vi "Config FX Extract.vi"(6 "Send Cmd Timout(ms)":u32=300, 8 "Error":errorcluster, 9 "CAN.Bus":string, 10 "HW Config":T1={"LiftHW Ver"=0, "CAN"={"ID Primary"=0, "Bus"="", "ID Follower"=0}, "Output"={"Type"=enum."Counter-Clockwise", "Neutral"=enum."Override to Coast", "Max"={"FWD"=1.0, "REV"=-1.0}, "Min"={"FWD"=0.0, "REV"=0.0}, "OL Ramp Rate (S)"=0.0, "Dead Band"=0.0}, "CLUp"={"Gains"={"P"=1.0, "I"=0.01, "D"=0.0, "F"=0.0}, "Error Allowed"={"High"=0.0, "Low"=0.0}, "I Zone"={"High"=10000.0, "Low"=-1000.0}, "Max Out"={"FWD"=1.0, "REV"=-1.0}, "Max I Accu"={"High"=10.0, "Low"=-10.0}, "CL Ramp Rate (S)"=0.0}, "MM"={"Cruise Velocity"=5000, "Acceleration"=5000}, "TravelLimits"={"Hard"={"FWD Switch Normal"=enum."Normally Open", "FWD On will Zero Encoder "=FALSE, "REV Switch Normal"=enum."Normally Open", "REV On will Zero Encoder "=FALSE}, "Soft"={"FWD"={"Enable"=FALSE, "Counts"=0}, "REV"={"Enable"=FALSE, "Counts"=0}}}, "Cancoder"={"ID"=0, "CW(t) CCW(f)"=TRUE, "Zero Offset"=0.0}, "CLDown"={"Gains"={"P"=1.0, "I"=0.01, "D"=0.0, "F"=0.0}, "Error Allowed"={"High"=0.0, "Low"=0.0}, "I Zone"={"High"=10000.0, "Low"=-1000.0}, "Max Out"={"FWD"=1.0, "REV"=-1.0}, "Max I Accu"={"High"=10.0, "Low"=-10.0}, "CL Ramp Rate (S)"=0.0}, "CurrentLimit"={"Enable"=FALSE, "Current Limit"=0.0, "Threshold Current"=0.0, "Threshold Time"=0.0}} {"CLDown"."Max I Accu"."Low" format="%#.8f"; "CLDown"."Max I Accu"."High" format="%#.8f"; "CLDown"."Gains"."F" format="%#.8f"; "CLDown"."Gains"."D" format="%#.8f"; "CLDown"."Gains"."I" format="%#.8f"; "CLDown"."Gains"."P" format="%#.8f"; "CLDown"."Error Allowed"."Low" format="%#.8f"; "CLDown"."Error Allowed"."High" format="%#.8f"; "CLDown"."I Zone"."Low" format="%#.8f"; "CLDown"."I Zone"."High" format="%#.8f"; "CLDown"."Max Out"."REV" format="%.2f"; "CLDown"."Max Out"."FWD" format="%.2f"; "TravelLimits"."Soft"."REV"."Counts" format="%#.0f"; "TravelLimits"."Soft"."FWD"."Counts" format="%#.0f"; "Output"."Min"."REV" format="%.2f"; "Output"."Min"."FWD" format="%.2f"; "Output"."Max"."REV" format="%.2f"; "Output"."Max"."FWD" format="%.2f"; "CLUp"."Max I Accu"."Low" format="%#.8f"; "CLUp"."Max I Accu"."High" format="%#.8f"; "CLUp"."Gains"."F" format="%#.8f"; "CLUp"."Gains"."D" format="%#.8f"; "CLUp"."Gains"."I" format="%#.8f"; "CLUp"."Gains"."P" format="%#.8f"; "CLUp"."Error Allowed"."Low" format="%#.8f"; "CLUp"."Error Allowed"."High" format="%#.8f"; "CLUp"."I Zone"."Low" format="%#.8f"; "CLUp"."I Zone"."High" format="%#.8f"; "CLUp"."Max Out"."REV" format="%.2f"; "CLUp"."Max Out"."FWD" format="%.2f"}, 11 "PhoenixMotorControlDevRef":T18={"DeviceStatus"={"status"=FALSE, "code"=0, "source"=""}, "Type"=enum."PWM", "PWM"={"PWM Channel"=enum."Invalid", "DeadBand"={"Name"="", "maxPositivePwm"=0, "minPositivePwm"=0, "centerPwm"=0, "maxNegativePwm"=0, "minNegativePwm"=0, "angularRange"=0}}, "CAN"={"Device Number"=0, "SetOutput VI Ref"=variant, "GetOutput VI Ref"=variant, "Enable VI Ref"=variant, "Disable VI Ref"=variant, "Data"=variant}, "Invert"=FALSE, "DIO PWM"={"PWM \"Enable\" Channel"=enum."Invalid", "DIOChannel"=enum."Invalid", "PWM Rate"=0.0}}) -> (0 "Error Out":errorcluster, 2 "HW Config Data Out":T1={"LiftHW Ver"=0, "CAN"={"ID Primary"=0, "Bus"="", "ID Follower"=0}, "Output"={"Type"=enum."Counter-Clockwise", "Neutral"=enum."Override to Coast", "Max"={"FWD"=1.0, "REV"=-1.0}, "Min"={"FWD"=0.0, "REV"=0.0}, "OL Ramp Rate (S)"=0.0, "Dead Band"=0.0}, "CLUp"={"Gains"={"P"=1.0, "I"=0.01, "D"=0.0, "F"=0.0}, "Error Allowed"={"High"=0.0, "Low"=0.0}, "I Zone"={"High"=10000.0, "Low"=-1000.0}, "Max Out"={"FWD"=1.0, "REV"=-1.0}, "Max I Accu"={"High"=10.0, "Low"=-10.0}, "CL Ramp Rate (S)"=0.0}, "MM"={"Cruise Velocity"=5000, "Acceleration"=5000}, "TravelLimits"={"Hard"={"FWD Switch Normal"=enum."Normally Open", "FWD On will Zero Encoder "=FALSE, "REV Switch Normal"=enum."Normally Open", "REV On will Zero Encoder "=FALSE}, "Soft"={"FWD"={"Enable"=FALSE, "Counts"=0}, "REV"={"Enable"=FALSE, "Counts"=0}}}, "Cancoder"={"ID"=0, "CW(t) CCW(f)"=TRUE, "Zero Offset"=0.0}, "CLDown"={"Gains"={"P"=1.0, "I"=0.01, "D"=0.0, "F"=0.0}, "Error Allowed"={"High"=0.0, "Low"=0.0}, "I Zone"={"High"=10000.0, "Low"=-1000.0}, "Max Out"={"FWD"=1.0, "REV"=-1.0}, "Max I Accu"={"High"=10.0, "Low"=-10.0}, "CL Ramp Rate (S)"=0.0}, "CurrentLimit"={"Enable"=FALSE, "Current Limit"=0.0, "Threshold Current"=0.0, "Threshold Time"=0.0}} {"CLDown"."Max I Accu"."Low" format="%#.8f"; "CLDown"."Max I Accu"."High" format="%#.8f"; "CLDown"."Gains"."F" format="%#.8f"; "CLDown"."Gains"."D" format="%#.8f"; "CLDown"."Gains"."I" format="%#.8f"; "CLDown"."Gains"."P" format="%#.8f"; "CLDown"."Error Allowed"."Low" format="%#.8f"; "CLDown"."Error Allowed"."High" format="%#.8f"; "CLDown"."I Zone"."Low" format="%#.8f"; "CLDown"."I Zone"."High" format="%#.8f"; "CLDown"."Max Out"."REV" format="%.2f"; "CLDown"."Max Out"."FWD" format="%.2f"; "TravelLimits"."Soft"."REV"."Counts" format="%#.0f"; "TravelLimits"."Soft"."FWD"."Counts" format="%#.0f"; "Output"."Min"."REV" format="%.2f"; "Output"."Min"."FWD" format="%.2f"; "Output"."Max"."REV" format="%.2f"; "Output"."Max"."FWD" format="%.2f"; "CLUp"."Max I Accu"."Low" format="%#.8f"; "CLUp"."Max I Accu"."High" format="%#.8f"; "CLUp"."Gains"."F" format="%#.8f"; "CLUp"."Gains"."D" format="%#.8f"; "CLUp"."Gains"."I" format="%#.8f"; "CLUp"."Gains"."P" format="%#.8f"; "CLUp"."Error Allowed"."Low" format="%#.8f"; "CLUp"."Error Allowed"."High" format="%#.8f"; "CLUp"."I Zone"."Low" format="%#.8f"; "CLUp"."I Zone"."High" format="%#.8f"; "CLUp"."Max Out"."REV" format="%.2f"; "CLUp"."Max Out"."FWD" format="%.2f"}, 3 "Module Azimuth Ref Out":T18)   [LabVIEW 2020, in "Lift_ACT.lvlib"]
uses:
  Lift_ACT.lvlib
  <vilib>/Rock Robotics/WPI/MotorControl/WPI_MotorControlDeviceRef.ctl
  <vilib>/Rock Robotics/WPI/MotorControl/WPI_MotorControlType.ctl
  <vilib>/Rock Robotics/SystemInterfaces/DIO/FPGA_DIOPWMChannel.ctl
  <vilib>/Rock Robotics/WPI/PWM/WPI_PWMDeadband.ctl
  <vilib>/Rock Robotics/SystemInterfaces/DIO/FPGA_DIOChannel.ctl
  Shared Code/TypeDefs/Cluster_Lift_Config HW Values.ctl
  Shared Code/TypeDefs/Cluser_CAN Follower Data.ctl
  Shared Code/TypeDefs/Cluster_Config Motor Output.ctl
  <vilib>/Rock Robotics/WPI/ThirdParty/Phoenix-LabVIEW/Motor Controller/Controls/CTRE_Phoenix_MotorControl_TalonFXInvertType.ctl
  <vilib>/Rock Robotics/WPI/ThirdParty/Phoenix-LabVIEW/Motor Controller/Controls/CTRE_Phoenix_MotorControl_NeutralMode.ctl
  Shared Code/TypeDefs/Cluster_FWD  REV Values.ctl
  Shared Code/TypeDefs/Cluster_PID Config.ctl
  Shared Code/TypeDefs/Cluster_PID Gains.ctl
  Shared Code/TypeDefs/Cluster_High-Low.ctl
  Shared Code/TypeDefs/Cluster_Motion Magic Parameters.ctl
  Shared Code/TypeDefs/Cluser_Limit Travel Config.ctl
  Shared Code/TypeDefs/Cluser_Hard Limits.ctl
  <vilib>/Rock Robotics/WPI/ThirdParty/Phoenix-LabVIEW/Motor Controller/Controls/CTRE_Phoenix_MotorControl_LimitSwitchNormal.ctl
  Shared Code/TypeDefs/Cluser_Config_Soft Limits.ctl
  Shared Code/TypeDefs/Cluser_Enable-Value I32.ctl
  Shared Code/TypeDefs/Cluster_Config_Cancoder Data.ctl
  Shared Code/TypeDefs/Cluser_Config_Current Limits.ctl
  <vilib>/Rock Robotics/WPI/ThirdParty/Phoenix-LabVIEW/Motor Controller/Controls/CTRE_Phoenix_MotorControl_TalonFXMotorControllerConfigurables.ctl
  <vilib>/Rock Robotics/WPI/ThirdParty/Phoenix-LabVIEW/Motor Controller/Controls/CTRE_Phoenix_MotorControl_BaseConfigurables.ctl
  <vilib>/Rock Robotics/WPI/ThirdParty/Phoenix-LabVIEW/Motor Controller/Controls/CTRE_Phoenix_MotorControl_VelocityMeasurementPeriod.ctl
  <vilib>/Rock Robotics/WPI/ThirdParty/Phoenix-LabVIEW/Motor Controller/Controls/CTRE_Phoenix_MotorControl_SlotStructure.ctl
  <vilib>/Rock Robotics/WPI/ThirdParty/Phoenix-LabVIEW/Motor Controller/Controls/CTRE_Phoenix_MotorControl_FilterStruct.ctl
  <vilib>/Rock Robotics/WPI/ThirdParty/Phoenix-LabVIEW/Motor Controller/Controls/CTRE_Phoenix_MotorControl_RemoteSourceType.ctl
  <vilib>/Rock Robotics/WPI/ThirdParty/Phoenix-LabVIEW/Controls/CTRE_Phoenix_CustomParamConfiguration.ctl
  <vilib>/Rock Robotics/WPI/ThirdParty/Phoenix-LabVIEW/Motor Controller/Controls/CTRE_Phoenix_MotorControl_FeedbackDevice_TalonFX.ctl
  <vilib>/Rock Robotics/WPI/ThirdParty/Phoenix-LabVIEW/Motor Controller/Controls/CTRE_Phoenix_MotorControl_LimitSwitchSource_Local.ctl
  <vilib>/Rock Robotics/WPI/ThirdParty/Phoenix-LabVIEW/Motor Controller/Controls/CTRE_Phoenix_MotorControl_SupplyCurrentLimitConfiguration.ctl
  <vilib>/Rock Robotics/WPI/ThirdParty/Phoenix-LabVIEW/Motor Controller/Controls/CTRE_Phoenix_MotorControl_StatorCurrentLimitConfiguration.ctl
  <vilib>/Rock Robotics/WPI/ThirdParty/Phoenix-LabVIEW/Motor Controller/Controls/CTRE_Phoenix_MotorControl_MotorCommutation_TalonFX.ctl
  <vilib>/Rock Robotics/WPI/ThirdParty/Phoenix-LabVIEW/CANCoder/Controls/CTRE_Phoenix_CANcoder_AbsoluteSensorRange.ctl
  <vilib>/Rock Robotics/WPI/ThirdParty/Phoenix-LabVIEW/CANCoder/Controls/CTRE_Phoenix_CANcoder_SensorInitializationStrategy.ctl
  <vilib>/Utility/Data Type/NI_Data Type.lvlib
panel:
  # "Tune Output\nto 1023 Max"
  # "Tune Output\nto 1023 Max"
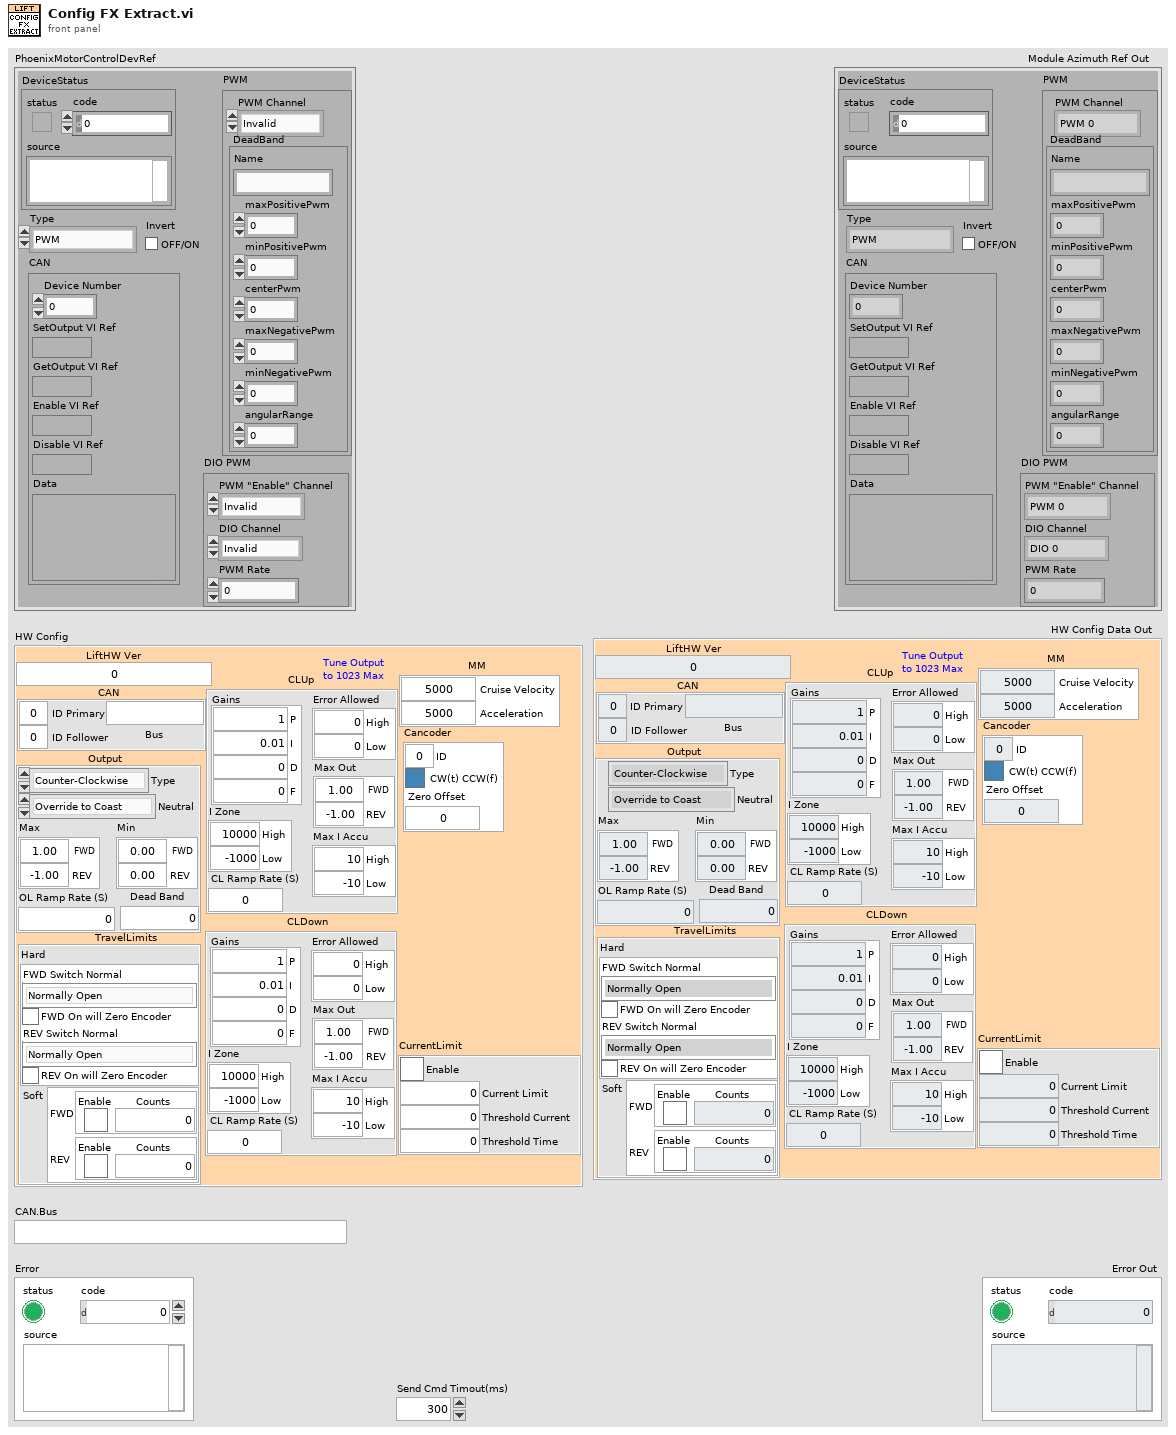
[diagram p1: front panel]
types:
  T1 = typedef "Cluster_Lift_Config HW Values.ctl" = cluster{"LiftHW Ver":u64, "CAN":T2, "Output":T3, "CLUp":T7, "MM":T10, "TravelLimits":T11, "Cancoder":T16, "CLDown":T7, "CurrentLimit":T17}
  T2 = typedef "Cluser_CAN Follower Data.ctl" = cluster{"ID Primary":u8, "Bus":string, "ID Follower":u8}
  T3 = typedef "Cluster_Config Motor Output.ctl" = cluster{"Type":T4, "Neutral":T5, "Max":T6, "Min":T6, "OL Ramp Rate (S)":dbl, "Dead Band":dbl}
  T4 = typedef "CTRE_Phoenix_MotorControl_TalonFXInvertType.ctl" = enum16{"Counter-Clockwise", "Clockwise"}
  T5 = typedef "CTRE_Phoenix_MotorControl_NeutralMode.ctl" = enum8{"EEPROMSetting", "Override to Coast", "Override to Brake"}
  T6 = typedef "Cluster_FWD  REV Values.ctl" = cluster{"FWD":dbl, "REV":dbl}
  T7 = typedef "Cluster_PID Config.ctl" = cluster{"Gains":T8, "Error Allowed":T9, "I Zone":T9, "Max Out":T6, "Max I Accu":T9, "CL Ramp Rate (S)":dbl}
  T8 = typedef "Cluster_PID Gains.ctl" = cluster{"P":dbl, "I":dbl, "D":dbl, "F":dbl}
  T9 = typedef "Cluster_High-Low.ctl" = cluster{"High":dbl, "Low":dbl}
  T10 = typedef "Cluster_Motion Magic Parameters.ctl" = cluster{"Cruise Velocity":i32, "Acceleration":i32}
  T11 = typedef "Cluser_Limit Travel Config.ctl" = cluster{"Hard":T12, "Soft":T14}
  T12 = typedef "Cluser_Hard Limits.ctl" = cluster{"FWD Switch Normal":T13, "FWD On will Zero Encoder ":bool, "REV Switch Normal":T13, "REV On will Zero Encoder ":bool}
  T13 = typedef "CTRE_Phoenix_MotorControl_LimitSwitchNormal.ctl" = enum16{"Normally Open", "Normally Closed", "Disabled"}
  T14 = typedef "Cluser_Config_Soft Limits.ctl" = cluster{"FWD":T15, "REV":T15}
  T15 = typedef "Cluser_Enable-Value I32.ctl" = cluster{"Enable":bool, "Counts":i32}
  T16 = typedef "Cluster_Config_Cancoder Data.ctl" = cluster{"ID":u8, "CW(t) CCW(f)":bool, "Zero Offset":dbl}
  T17 = typedef "Cluser_Config_Current Limits.ctl" = cluster{"Enable":bool, "Current Limit":dbl, "Threshold Current":dbl, "Threshold Time":dbl}
  T18 = typedef "WPI_MotorControlDeviceRef.ctl" = cluster{"DeviceStatus":errorcluster, "Type":T19, "PWM":cluster{"PWM Channel":T20, "DeadBand":T21}, "CAN":cluster{"Device Number":u8, "SetOutput VI Ref":variant, "GetOutput VI Ref":variant, "Enable VI Ref":variant, "Disable VI Ref":variant, "Data":variant}, "Invert":bool, "DIO PWM":cluster{"PWM \"Enable\" Channel":T20, "DIOChannel":T22, "PWM Rate":dbl}}
  T19 = typedef "WPI_MotorControlType.ctl" = enum16{"PWM", "CAN", "DIO PWM"}
  T20 = typedef "FPGA_DIOPWMChannel.ctl" = enum8{"PWM 0", "PWM 1", "PWM 2", "PWM 3", "PWM 4", "PWM 5", "PWM 6", "PWM 7", "PWM 8", "PWM 9", "PWM MXP 0", "PWM MXP 1", "PWM MXP 2", "PWM MXP 3", "PWM MXP 4", "PWM MXP 5", "PWM MXP 6", "PWM MXP 7", "PWM MXP 8", "PWM MXP 9", "Invalid"}
  T21 = typedef "WPI_PWMDeadband.ctl" = cluster{"Name":string, "maxPositivePwm":i32, "minPositivePwm":i32, "centerPwm":i32, "maxNegativePwm":i32, "minNegativePwm":i32, "angularRange":u16}
  T22 = typedef "FPGA_DIOChannel.ctl" = enum8{"DIO 0", "DIO 1", "DIO 2", "DIO 3", "DIO 4", "DIO 5", "DIO 6", "DIO 7", "DIO 8", "DIO 9", "DIO MXP 0", "DIO MXP 1", "DIO MXP 2", "DIO MXP 3", "DIO MXP 4", "DIO MXP 5", "DIO MXP 6", "DIO MXP 7", "DIO MXP 8", "DIO MXP 9", "DIO MXP 10", "DIO MXP 11", "DIO MXP 12", "DIO MXP 13", "DIO MXP 14", "DIO MXP 15", "SPI Port CS1", "SPI Port CS2", "SPI Port CS3", "SPI Port MISO", "SPI Port MOSI", "Invalid"}
  T23 = typedef "CTRE_Phoenix_MotorControl_TalonFXMotorControllerConfigurables.ctl" = cluster{"Base Configurables":T24, "primaryPID":cluster{"selectedFeedbackCoefficient":dbl, "selectedFeedbackSensor":T30}, "auxiliaryPID":cluster{"selectedFeedbackCoefficient":dbl, "selectedFeedbackSensor":T30}, "forwardLimitSwitchNormal":T13, "reverseLimitSwitchNormal":T13, "forwardLimitSwitchDeviceID":i32, "reverseLimitSwitchDeviceID":i32, "forwardLimitSwitchSource":T31, "reverseLimitSwitchSource":T31, "sum0Term":T30, "sum1Term":T30, "diff0Term":T30, "diff1Term":T30, "Supply Current Limit Configuration":T32, "Stator Current Limit Configuration":T33, "Motor Commutation":T34, "Absolute Sensor Range":T35, "Integrated Sensor Offset (Degrees)":dbl, "Sensor Initialization Strategy":T36}
  T24 = typedef "CTRE_Phoenix_MotorControl_BaseConfigurables.ctl" = cluster{"openLoopRamp":dbl, "closedLoopRamp":dbl, "peakOutputForward":dbl, "peakOutputReverse":dbl, "nominalOutputForward":dbl, "nominalOutputReverse":dbl, "neutralDeadband":dbl, "voltageCompSaturation":dbl, "voltageMeasurementFilter":i32, "velocityMeasurementPeriod":T25, "velocityMeasurementWindow":i32, "forwardSoftLimitThreshold":i32, "reverseSoftLimitThreshold":i32, "forwardSoftLimitEnable":bool, "reverseSoftLimitEnable":bool, "slot0":T26, "slot1":T26, "slot2":T26, "slot3":T26, "auxPIDPolarity":bool, "remoteFilter0":T27, "remoteFilter1":T27, "motionCruiseVelocity":i32, "motionAcceleration":i32, "motionProfileTrajectoryPeriod":i32, "feedbackNotContinuous":bool, "remoteSensorClosedLoopDisableNeutralOnLOS":bool, "clearPositionOnLimitF":bool, "clearPositionOnLimitR":bool, "clearPositionOnQuadIdx":bool, "limitSwitchDisableNeutralOnLOS":bool, "softLimitDisableNeutralOnLOS":bool, "pulseWidthPeriod_EdgesPerRot":i32, "pulseWidthPeriod_FilterWindowSz":i32, "customParam":T29, "trajectoryInterpolationEnable":bool}
  T25 = typedef "CTRE_Phoenix_MotorControl_VelocityMeasurementPeriod.ctl" = u16
  T26 = typedef "CTRE_Phoenix_MotorControl_SlotStructure.ctl" = cluster{"P":dbl, "I":dbl, "D":dbl, "F":dbl, "integralZone":dbl, "allowableClosedLoopError":i32, "maxIntegralAccumulator":dbl, "closedLoopPeakOutput":dbl, "closedLoopPeriod":i32}
  T27 = typedef "CTRE_Phoenix_MotorControl_FilterStruct.ctl" = cluster{"remoteSensorDeviceID":u8, "remoteSensorSource":T28}
  T28 = typedef "CTRE_Phoenix_MotorControl_RemoteSourceType.ctl" = enum16{"Off", "Talon SRX Selected Sensor", "Pigeon IMU Yaw", "Pigeon IMU Pitch", "Pigeon IMU Roll", "CANifier Quadrature", "CANifier PWM Input 0", "CANifier PWM Input 1", "CANifier PWM Input 2", "CANifier PWM Input 3", "Gadgeteer Pigeon Yaw", "Gadgeteer Pigeon Pitch", "Gadgeteer Pigeon Roll", "CANCoder"}
  T29 = typedef "CTRE_Phoenix_CustomParamConfiguration.ctl" = cluster{"customParam0":i32, "customParam1":i32}
  T30 = typedef "CTRE_Phoenix_MotorControl_FeedbackDevice_TalonFX.ctl" = i8
  T31 = typedef "CTRE_Phoenix_MotorControl_LimitSwitchSource_Local.ctl" = enum16{"Feedback Connector", "Remote Talon SRX", "Remote CANifier", "Deactivated"}
  T32 = typedef "CTRE_Phoenix_MotorControl_SupplyCurrentLimitConfiguration.ctl" = cluster{"Enable?":bool, "Current Limit":dbl, "Threshold Current":dbl, "Threshold Time":dbl}
  T33 = typedef "CTRE_Phoenix_MotorControl_StatorCurrentLimitConfiguration.ctl" = cluster{"Enable?":bool, "Current Limit":dbl, "Threshold Current":dbl, "Threshold Time":dbl}
  T34 = typedef "CTRE_Phoenix_MotorControl_MotorCommutation_TalonFX.ctl" = enum16{"Trapezoidal"}
  T35 = typedef "CTRE_Phoenix_CANcoder_AbsoluteSensorRange.ctl" = enum16{"Unsigned [0 to 360)", "Signed [-180 to +180)"}
  T36 = typedef "CTRE_Phoenix_CANcoder_SensorInitializationStrategy.ctl" = enum16{"Boot To Zero", "Boot To Absolute Position"}
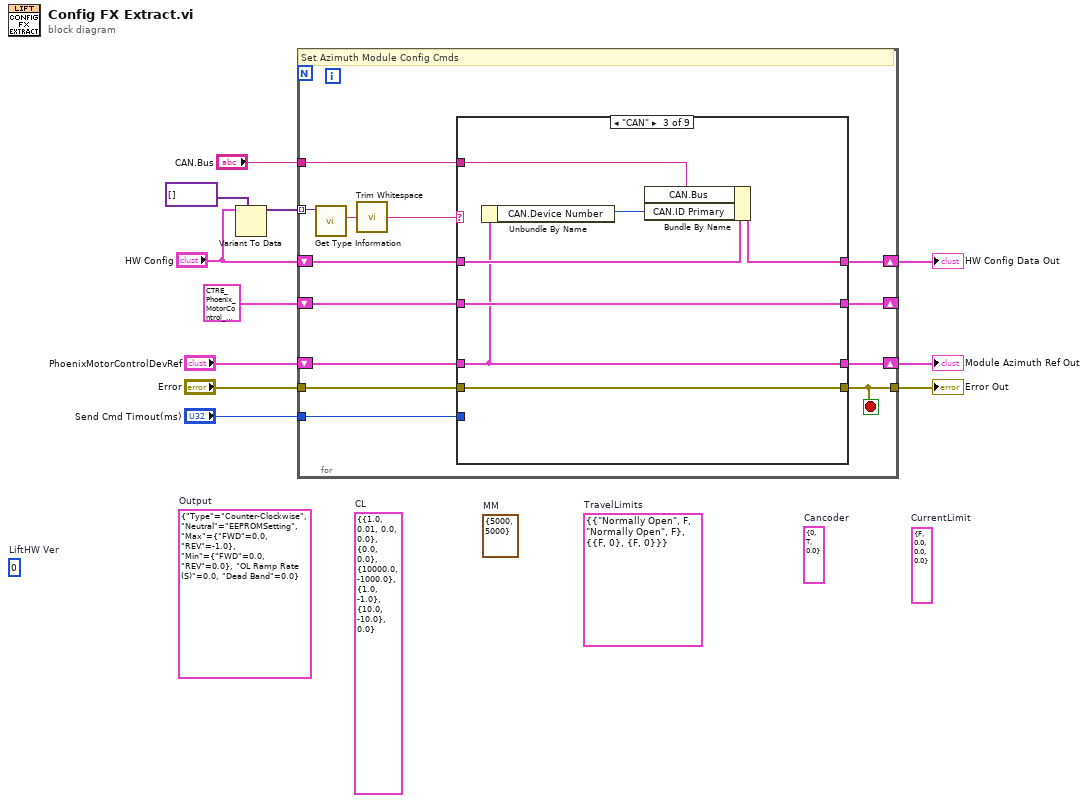
[diagram p0: block diagram]
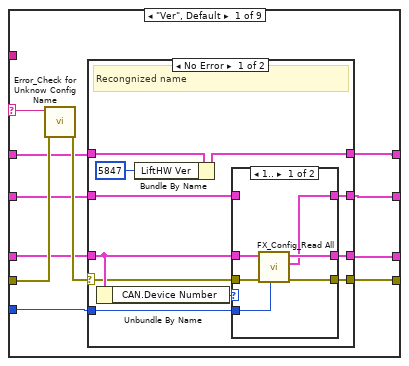
[diagram p2: hidden frame]
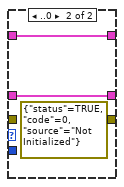
[diagram p3: hidden frame]
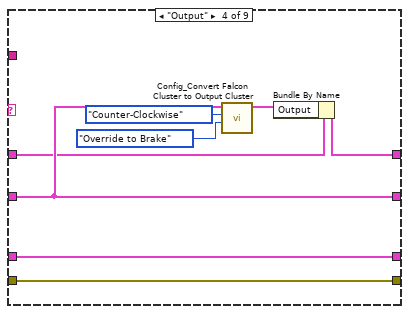
[diagram p6: hidden frame]
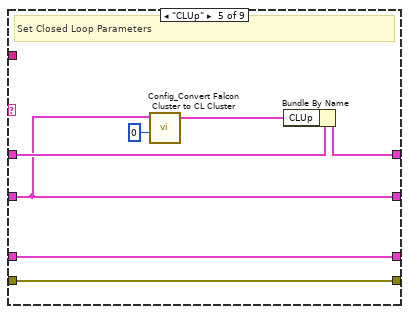
[diagram p7: hidden frame]
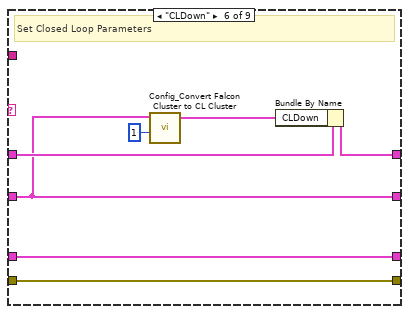
[diagram p8: hidden frame]
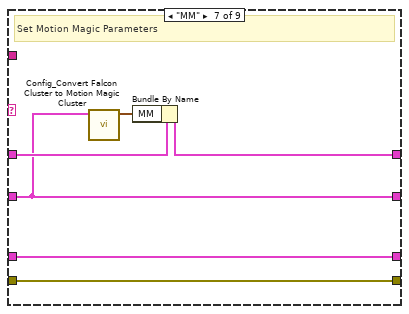
[diagram p9: hidden frame]
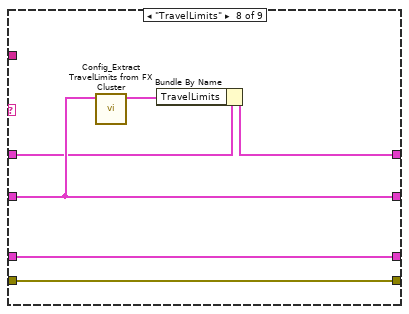
[diagram p10: hidden frame]
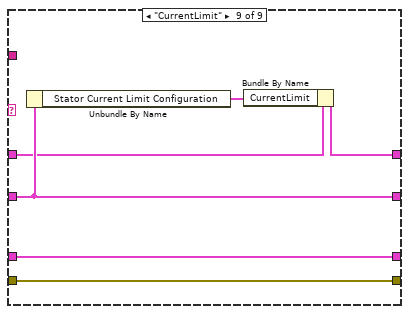
[diagram p11: hidden frame]
diagram:
  (unwired) T17 {"Enable"=FALSE, "Current Limit"=0.0, "Threshold Current"=0.0, "Threshold Time"=0.0}  # CurrentLimit
  (unwired) T16 {"ID"=0, "CW(t) CCW(f)"=TRUE, "Zero Offset"=0.0}  # Cancoder
  (unwired) T10 {"Cruise Velocity"=5000, "Acceleration"=5000}  # MM
  (unwired) T11 {"Hard"={"FWD Switch Normal"=enum."Normally Open", "FWD On will Zero Encoder "=FALSE, "REV Switch Normal"=enum."Normally Open", "REV On will Zero Encoder "=FALSE}, "Soft"={"FWD"={"Enable"=FALSE, "Counts"=0}, "REV"={"Enable"=FALSE, "Counts"=0}}}  # TravelLimits
  (unwired) T7 {"Gains"={"P"=1.0, "I"=0.01, "D"=0.0, "F"=0.0}, "Error Allowed"={"High"=0.0, "Low"=0.0}, "I Zone"={"High"=10000.0, "Low"=-1000.0}, "Max Out"={"FWD"=1.0, "REV"=-1.0}, "Max I Accu"={"High"=10.0, "Low"=-10.0}, "CL Ramp Rate (S)"=0.0}  # CL
  (unwired) T3 {"Type"=enum."Counter-Clockwise", "Neutral"=enum."EEPROMSetting", "Max"={"FWD"=0.0, "REV"=-1.0}, "Min"={"FWD"=0.0, "REV"=0.0}, "OL Ramp Rate (S)"=0.0, "Dead Band"=0.0}  # Output
  (unwired) u64 0  # LiftHW Ver
  n1 = Variant To Data(type=variant[] [], Variant="HW Config") -> (data=w2:variant[])  [unwired: 1 in, 1 out]
  n2 = for {
    tunnel: "Send Cmd Timout(ms)" -> [w23]
    shift-right: [w24] -> w11
    shift-left: "PhoenixMotorControlDevRef" -> [w21]
    tunnel: w2 -> [w20] mode=indexing
    tunnel: "Error" -> [w12]
    tunnel: [w18] -> w10
    shift-right: [w19] -> w4
    shift-left: "HW Config" -> [w22]
    shift-right: [w17] -> _
    shift-left: T23 {"Base Configurables"={"openLoopRamp"=0.0, "closedLoopRamp"=0.0, "peakOutputForward"=1.0, "peakOutputReverse"=-1.0, "nominalOutputForward"=0.0, "nominalOutputReverse"=0.0, "neutralDeadband"=0.04, "voltageCompSaturation"=0.0, "voltageMeasurementFilter"=32, "velocityMeasurementPeriod"=100, "velocityMeasurementWindow"=64, "forwardSoftLimitThreshold"=0, "reverseSoftLimitThreshold"=0, "forwardSoftLimitEnable"=FALSE, "reverseSoftLimitEnable"=FALSE, "slot0"={"P"=0.0, "I"=0.0, "D"=0.0, "F"=0.0, "integralZone"=0.0, "allowableClosedLoopError"=0, "maxIntegralAccumulator"=0.0, "closedLoopPeakOutput"=1.0, "closedLoopPeriod"=1}, "slot1"={"P"=0.0, "I"=0.0, "D"=0.0, "F"=0.0, "integralZone"=0.0, "allowableClosedLoopError"=0, "maxIntegralAccumulator"=0.0, "closedLoopPeakOutput"=1.0, "closedLoopPeriod"=1}, "slot2"={"P"=0.0, "I"=0.0, "D"=0.0, "F"=0.0, "integralZone"=0.0, "allowableClosedLoopError"=0, "maxIntegralAccumulator"=0.0, "closedLoopPeakOutput"=1.0, "closedLoopPeriod"=1}, "slot3"={"P"=0.0, "I"=0.0, "D"=0.0, "F"=0.0, "integralZone"=0.0, "allowableClosedLoopError"=0, "maxIntegralAccumulator"=0.0, "closedLoopPeakOutput"=1.0, "closedLoopPeriod"=1}, "auxPIDPolarity"=FALSE, "remoteFilter0"={"remoteSensorDeviceID"=0, "remoteSensorSource"=enum."Off"}, "remoteFilter1"={"remoteSensorDeviceID"=0, "remoteSensorSource"=enum."Off"}, "motionCruiseVelocity"=0, "motionAcceleration"=0, "motionProfileTrajectoryPeriod"=0, "feedbackNotContinuous"=FALSE, "remoteSensorClosedLoopDisableNeutralOnLOS"=FALSE, "clearPositionOnLimitF"=FALSE, "clearPositionOnLimitR"=FALSE, "clearPositionOnQuadIdx"=FALSE, "limitSwitchDisableNeutralOnLOS"=FALSE, "softLimitDisableNeutralOnLOS"=FALSE, "pulseWidthPeriod_EdgesPerRot"=1, "pulseWidthPeriod_FilterWindowSz"=1, "customParam"={"customParam0"=0, "customParam1"=0}, "trajectoryInterpolationEnable"=TRUE}, "primaryPID"={"selectedFeedbackCoefficient"=1.0, "selectedFeedbackSensor"=1}, "auxiliaryPID"={"selectedFeedbackCoefficient"=1.0, "selectedFeedbackSensor"=1}, "forwardLimitSwitchNormal"=enum."Normally Open", "reverseLimitSwitchNormal"=enum."Normally Open", "forwardLimitSwitchDeviceID"=0, "reverseLimitSwitchDeviceID"=0, "forwardLimitSwitchSource"=enum."Feedback Connector", "reverseLimitSwitchSource"=enum."Feedback Connector", "sum0Term"=1, "sum1Term"=1, "diff0Term"=1, "diff1Term"=1, "Supply Current Limit Configuration"={"Enable?"=FALSE, "Current Limit"=0.0, "Threshold Current"=0.0, "Threshold Time"=0.0}, "Stator Current Limit Configuration"={"Enable?"=FALSE, "Current Limit"=0.0, "Threshold Current"=0.0, "Threshold Time"=0.0}, "Motor Commutation"=enum."Trapezoidal", "Absolute Sensor Range"=enum."Unsigned [0 to 360)", "Integrated Sensor Offset (Degrees)"=0.0, "Sensor Initialization Strategy"=enum."Boot To Zero"} ("Talon FX Configurables") -> [w16]
    tunnel: "CAN.Bus" -> [w13]
    stop <- w18 stop-if-true
    # "Set Azimuth Module Config Cmds"
    n3 = call <vilib>:"Get Type Information.vi"("variant"=w20) -> ("name"=w15:string)  [unwired: 6 in, 4 out]
    n4 = call <vilib>:"Trim Whitespace.vi"("string"=w15) -> ("trimmed string"=w14:string)  [unwired: 1 in]
    n5 = case shown="\"CAN\"" w14 {
      selector: w14 -> [w27 _ _ _ _ _ _ _ _]
      tunnel: [w33 w60 w70 w78 w84 w91 w95 w104 w109] -> w18
      tunnel: w23 -> [w25 _ _ _ _ _ _ _ _]
      tunnel: w21 -> [w30 w63 w65 w77 w85 w92 w96 w103 w110]
      tunnel: [w32 w63 w65 w77 w85 w92 w96 w103 w110] -> w24
      tunnel: w22 -> [w28 w62 w67 w71 w83 w90 w97 w100 w105]
      tunnel: [w26 w62 w68 w72 w82 w89 w98 w101 w106] -> w19
      tunnel: [w31 w61 w69 w76 w79 w86 w94 w102 w107] -> w17
      tunnel: w16 -> [w29 w61 w69 w76 w79 w86 w94 w102 w107]
      tunnel: w13 -> [_ _ w66 _ _ _ _ _ _]
      tunnel: w12 -> [w34 w60 w70 w78 w84 w91 w95 w104 w109]
      frame "Ver", Default {
        n6 = call "Error_Check for Unknow Config Name.vi"("error in (no error)"=w34, "Config Name"=w27) -> ("error out"=w35:errorcluster)  [unwired: 9 in]
        n7 = case shown="No Error" w35 {
          selector: w35 -> [w36 w57]
          tunnel: [w45 w57] -> w33
          tunnel: w30 -> [w44 w56]
          tunnel: [w43 w56] -> w32
          tunnel: [w42 w58] -> w31
          tunnel: w25 -> [w41 _]
          tunnel: w29 -> [w40 w58]
          tunnel: [w38 w59] -> w26
          tunnel: w28 -> [w37 w59]
          frame No Error {
            # "Recongnized name"
            n8 = Unbundle By Name(w44) -> ("CAN.Device Number"=w46:u8)
            n9 = Bundle By Name(cluster=w37, "LiftHW Ver"=u64 5847 ("ModuleAzimuth Ver")) -> (w38:T1)
            n10 = case shown="1.." w46 {
              tunnel: [w50 errorcluster {"status"=TRUE, "code"=0, "source"="Not Initialized"} ("error out")] -> w45
              tunnel: w44 -> [w52 w54]
              tunnel: [w49 w54] -> w43
              tunnel: [w48 w53] -> w42
              tunnel: w36 -> [w51 _]
              tunnel: w41 -> [w47 _]
              tunnel: w40 -> [_ w53]
              frame 1.. {
                n11 = call "FX_Config_Read All.vi"("Send Cmd Timout(ms)"=w47, "Error"=w51, "PhoenixMotorControlDevRef"=w52) -> ("Error Out"=w50:errorcluster, "FX Config Out"=w48:T23, "Ref Out"=w49:T18)  [unwired: 6 in]
              }
              frame ..0 {
              }
            }
          }
          frame Error {
            # "Unrecognized name"
          }
        }
      }
      frame "Cancoder" {
      }
      frame "CAN" {
        n12 = Unbundle By Name(w65) -> ("CAN.Device Number"=w64:u8)
        n13 = Bundle By Name(cluster=w67, "CAN.Bus"=w66, "CAN.ID Primary"=w64) -> (w68:T1)
      }
      frame "Output" {
        n14 = call "Config_Convert Falcon Cluster to Output Cluster.vi"("Neutral Mode"=CTRE_Phoenix_MotorControl_NeutralMode."Override to Brake", "Rotation Type"=CTRE_Phoenix_MotorControl_TalonFXInvertType."Counter-Clockwise", "Talon FX Configurables"=w76) -> ("Motor Output Out"=w73:T3)  [unwired: 8 in]
        n15 = Bundle By Name(cluster=w71, "Output"=w73) -> (w72:T1)
      }
      frame "CLUp" {
        # "Set Closed Loop Parameters"
        n16 = call "Config_Convert Falcon Cluster to CL Cluster.vi"("Slot"=0, "Talon FX Configurables"=w79) -> ("CL"=w81:T7)  [unwired: 8 in, 1 out]
        n17 = Bundle By Name(cluster=w83, "CLUp"=w81) -> (w82:T1)
      }
      frame "CLDown" {
        # "Set Closed Loop Parameters"
        n18 = call "Config_Convert Falcon Cluster to CL Cluster.vi"("Slot"=1, "Talon FX Configurables"=w86) -> ("CL"=w88:T7)  [unwired: 8 in, 1 out]
        n19 = Bundle By Name(cluster=w90, "CLDown"=w88) -> (w89:T1)
      }
      frame "MM" {
        # "Set Motion Magic Parameters"
        n20 = call "Config_Convert Falcon Cluster to Motion Magic Cluster.vi"("Talon FX Configurables"=w94) -> ("MM"=w93:T10)  [unwired: 10 in]
        n21 = Bundle By Name(cluster=w97, "MM"=w93) -> (w98:T1)
      }
      frame "TravelLimits" {
        n22 = call "Config_Extract TravelLimits from FX Cluster.vi"("Talon FX Configurables"=w102) -> ("Limits Out"=w99:T11)  [unwired: 10 in]
        n23 = Bundle By Name(cluster=w100, "TravelLimits"=w99) -> (w101:T1)
      }
      frame "CurrentLimit" {
        n24 = Unbundle By Name(w107) -> ("Stator Current Limit Configuration"=w108:T33)
        n25 = Bundle By Name(cluster=w105, "CurrentLimit"=w108) -> (w106:T1)
      }
    }
  }
  "Module Azimuth Ref Out" <- w11
  "Error Out" <- w10
  "HW Config Data Out" <- w4
